vi "white two sec run.vi"() -> ()   [LabVIEW 2010]
uses:
  <vilib>/NXT/Subs/MotorOutput.ctl
  <vilib>/NXT/Block Support/NXT_InputPort.ctl
  <vilib>/NXT/Dual Mode Library/Motors/MotorOn.vi
  <vilib>/NXT/Dual Mode Library/Waits/Wait_Num.vi
panel:
  in  "Output Port (All Ports)":T1=3 items=["Port A", "Port B", "Port C", "All Ports"]
  in  "빛 센서 포트(Port 4)":T2=2 caption="Port (Port 3)" items=["Port 1", "Port 2", "Port 3", "Port 4"]
  in  "회전 각도 2":i32=180
  in  "회전 각도 1":i32=180
  in  "회전 포트 1":T1=3 items=["Port A", "Port B", "Port C", "All Ports"]
  in  "회전 포트 2":T1=3 items=["Port A", "Port B", "Port C", "All Ports"]
  in  "후진 시간":sgl=1.0
  in  "Power (75)":i32=75
  in  "후진 포트":T1=3 items=["Port A", "Port B", "Port C", "All Ports"]
  in  "stop":bool
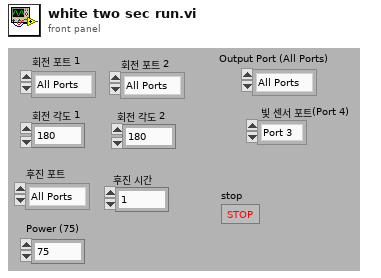
[diagram p1: front panel]
types:
  T1 = typedef "MotorOutput.ctl" = u8
  T2 = typedef "NXT_InputPort.ctl" = u8
  T3 = typedef "LVHSConnector.ctl" = cluster{"error":errorcluster, "address":string, "NXT #":i32, "Show Error":bool, "Connection":u16}
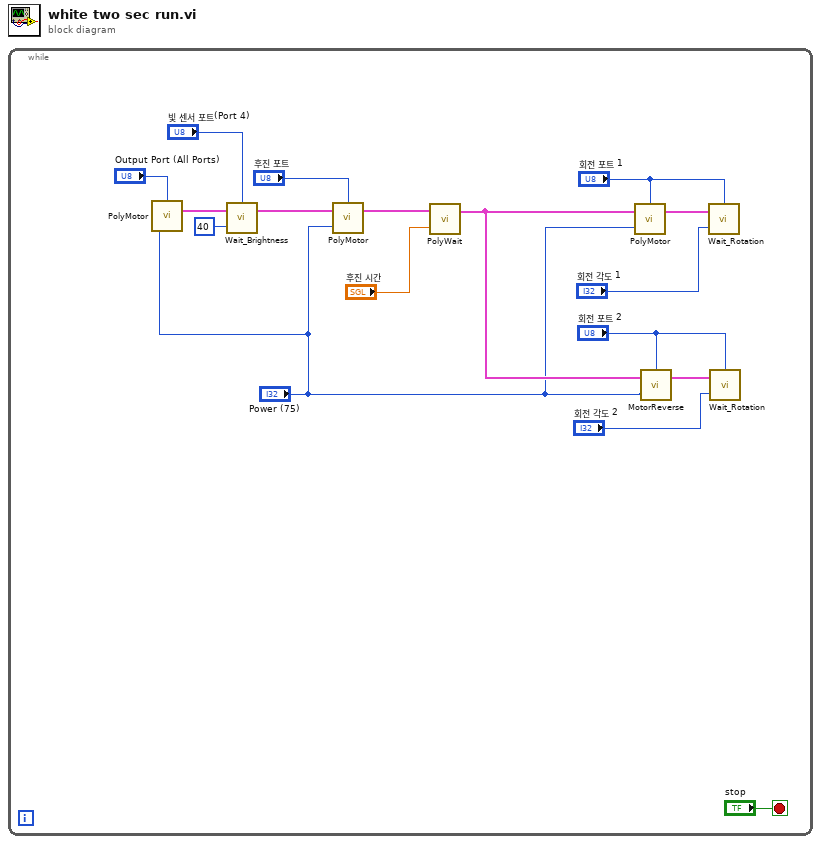
[diagram p0: block diagram]
diagram:
  n1 = while {
    stop <- "stop" stop-if-true
    n2 = call-poly <vilib>:"PolyMotor.vi"("Power (75)"="Power (75)", "Output Port (All Ports)"="Output Port (All Ports)") -> ("NXT"=w2:T3)  [unwired: 2 in]
    n3 = call <vilib>:"Wait_Brightness.vi"("Brightness (40)"=u8 40, "NXT"=w2, "Port (Port 3)"="빛 센서 포트(Port 4)") -> ("NXT"=w3:T3)  [unwired: 1 in]
    n4 = call-poly <vilib>:"PolyMotor.vi"("Power (75)"="Power (75)", "NXT"=w3, "Output Port (All Ports)"="후진 포트") -> ("NXT"=w16:T3)  [unwired: 1 in]
    n5 = call-poly <vilib>:"PolyWait.vi"("Time (sec)"="후진 시간", "NXT"=w16) -> ("NXT"=w14:T3)  [unwired: 2 in]
    n6 = call-poly <vilib>:"PolyMotor.vi"("Power (75)"="Power (75)", "NXT"=w14, "Output Port (All Ports)"="회전 포트 1") -> ("NXT"=w15:T3)  [unwired: 1 in]
    n7 = call <vilib>:"MotorReverse.vi"("Power (75)"="Power (75)", "NXT"=w14, "Output Port (All Ports)"="회전 포트 2") -> ("NXT"=w13:T3)  [unwired: 1 in]
    n8 = call <vilib>:"Wait_Rotation.vi"("Position Change (180)"="회전 각도 1", "NXT"=w15, "Port (Port A)"="회전 포트 1") -> ()  [unwired: 1 in, 1 out]
    n9 = call <vilib>:"Wait_Rotation.vi"("Position Change (180)"="회전 각도 2", "NXT"=w13, "Port (Port A)"="회전 포트 2") -> ()  [unwired: 1 in, 1 out]
  }
